vi "Digital - Continuous Output.vi"() -> ()   [LabVIEW 2020]
doc: "This example demonstrates how to continuously re-generate digital output data. That output is hardware timed, so each sample is output on the next tick of the sample clock.\n\nSome hardware (e.g. M Series DAQ) must use an external sample clock for digital tasks. To view a complete list of available sample clock sources, consult the Device Routes table in Measurement and Automation Explorer.\n\nFor instructions on how to connect your signals to the DAQ device, refer to your device documentation."
uses:
  <vilib>/Utility/error.llb/DialogType.ctl
  <vilib>/DAQmx/write.llb/DAQmx Write (Digital 1D U32 1Chan NSamp).vi
  <vilib>/DAQmx/create/channels.llb/DAQmx Create Channel (DO-Digital Output).vi
  <vilib>/DAQmx/configure/timing.llb/DAQmx Timing (Sample Clock).vi
  <vilib>/DAQmx/configure/trigger.llb/DAQmx Start Trigger (Digital Edge).vi
  <vilib>/DAQmx/configure/trigger.llb/DAQmx Start Trigger (Time).vi
  <vilib>/DAQmx/miscellaneous.llb/DAQmx Fill In Error Info.vi
  <resource>/objmgr/daqmx.rc
panel:
  in  "Frequency of Steps":dbl
  in  "Line(s)":tag="Dev1/port0/line0:7"
  in  "Stop":bool
  in  "Output Array":u32[](array[numeric])=[1, 2, 4, 8, 16, 32, 64, 128]
  in  "Trigger Type":T1(tab)
  in  "Edge":i32(ring)=10280 items=["Rising"=10280, "Falling"=10171]
  in  "Digital Trigger Source":tag="PFI1"
  in  "When":timestamp
  in  "Select Time\nManually":bool
  in  "Number of Samples":i32=1000
  in  "Sample Rate":dbl=1000.0
  in  "Sample Clock Source":tag="PFI0"
  out "Actual Sample Rate":dbl=1000.0 format="%0.2f"
  # "Channel Settings"
  # "Data to Write"
  # "Timing and Buffer Settings"
  # "Trigger Settings"
  # "To configure and use a start trigger you must have the necessary tab selected above.  Not all hardware supports triggering--refer to your device documentation for more info."
  # "If time is not manually set, task will begin after 10 seconds"
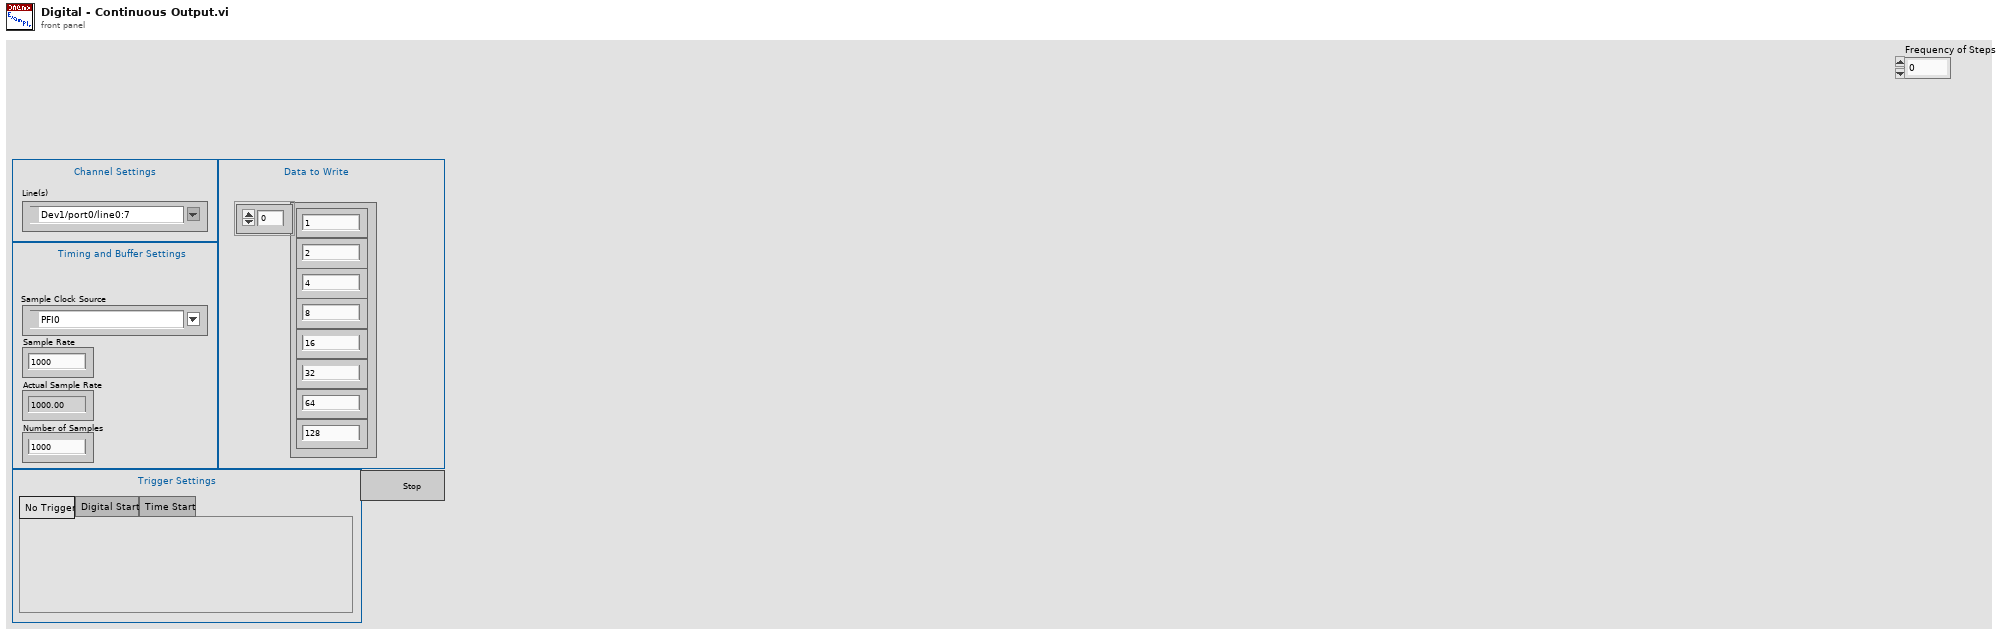
[diagram p1: front panel]
types:
  T1 = enum32{"No Trigger", "Digital Start", "Time Start"}
  T2 = typedef "DialogType.ctl" = u16
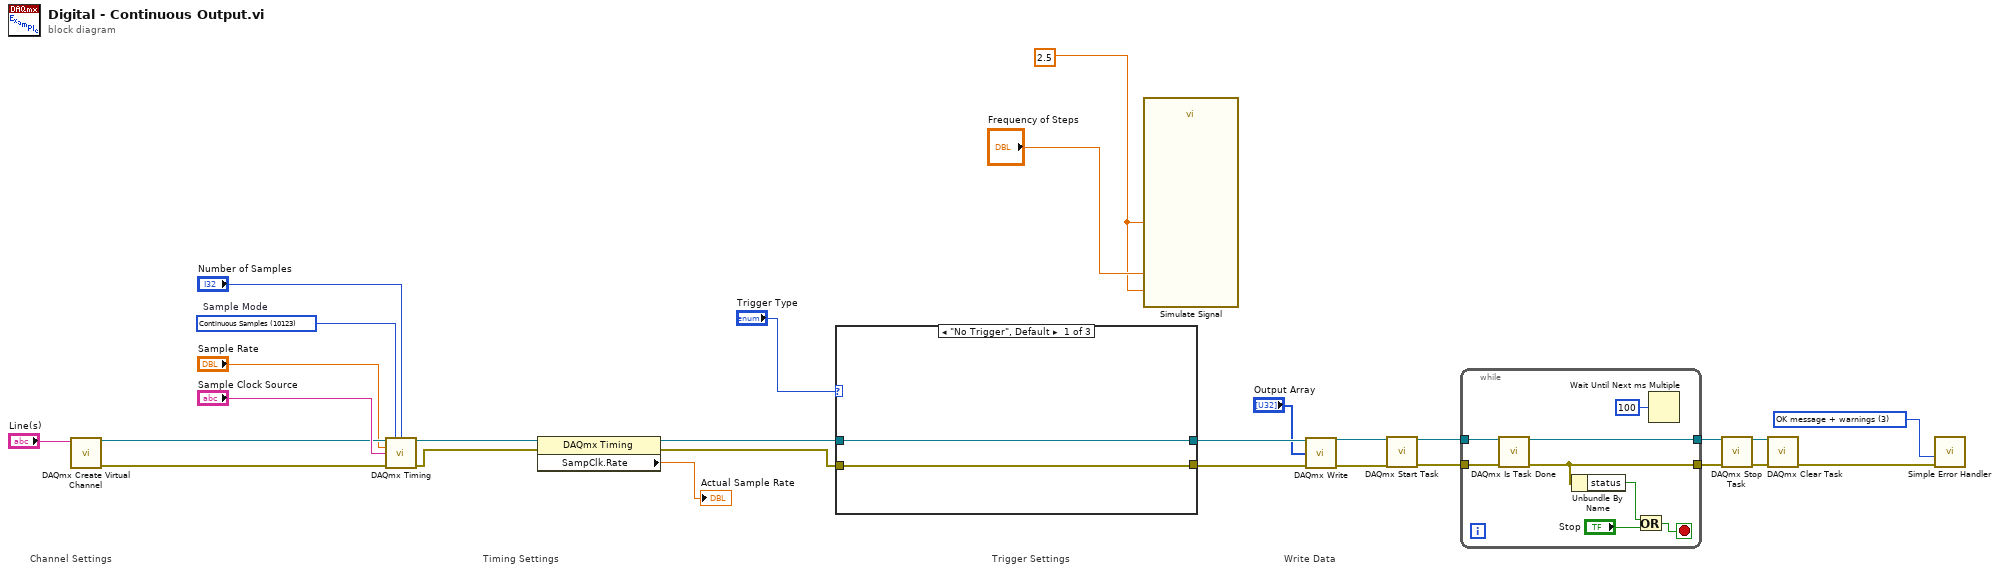
[diagram p0: block diagram]
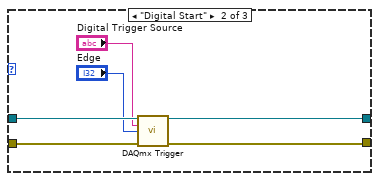
[diagram p2: hidden frame]
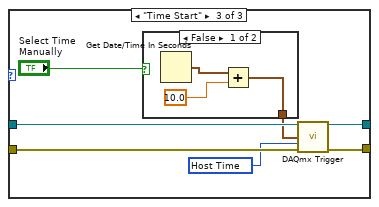
[diagram p3: hidden frame]
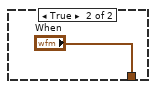
[diagram p4: hidden frame]
diagram:
  w1 = 2.5
  w3 = T2 3 items=["no dialog", "OK message", "continue or stop message", "OK message + warnings", "continue/stop + warnings"] ("type of dialog (OK msg:1)")
  w21 = 10123 items=["Finite Samples"=10178, "Continuous Samples"=10123, "Hardware Timed Single Point"=12522]  # Sample Mode
  # "Trigger Settings"
  # "Timing Settings"
  # "Write Data"
  # "Channel Settings"
  n1 = call-poly <vilib>:"DAQmx Create Virtual Channel.vi"("lines"="Line(s)") -> ("task out"=w25:refnum<k21>, "error out"=w24:errorcluster)  [unwired: 13 in]
  n2 = call-poly <vilib>:"DAQmx Timing.vi"("task/channels in"=w25, "sample mode"=w21, "samples per channel"="Number of Samples", "rate"="Sample Rate", "source"="Sample Clock Source", "error in"=w24) -> ("task out"=w20:refnum<k21>, "error out"=w19:errorcluster)  [unwired: 8 in]
  n3 = property class="DAQmx Timing"(reference=w20, error in=w19) -> (reference out=w17:refnum<k21>, error out=w16:errorcluster, "SampClk.Rate"=→"Actual Sample Rate":dbl)
  n4 = case shown="\"No Trigger\", Default" "Trigger Type" {
    tunnel: w17 -> [w30 w36 w43]
    tunnel: w16 -> [w29 w35 w42]
    tunnel: [w30 w34 w41] -> w15
    tunnel: [w29 w33 w40] -> w14
    frame "No Trigger", Default {
    }
    frame "Digital Start" {
      n5 = call-poly <vilib>:"DAQmx Trigger.vi"("task/channels in"=w36, "source"="Digital Trigger Source", "edge"="Edge", "error in"=w35) -> ("task out"=w34:refnum<k21>, "error out"=w33:errorcluster)  [unwired: 10 in]
    }
    frame "Time Start" {
      w37 = 16126 items=["Host Time"=16126, "I/O Device Time"=16127] ("timescale")
      n6 = case shown="False" "Select Time\nManually" {
        tunnel: [w45 "When"] -> w38
        frame False {
          n7 = Get Date/Time In Seconds() -> (seconds since 1Jan1904=w46:timestamp)
          n8 = Add(x=w46, y=10.0) -> (x+y=w45:timestamp)
        }
        frame True {
        }
      }
      n9 = call-poly <vilib>:"DAQmx Trigger.vi"("task/channels in"=w43, "when"=w38, "timescale"=w37, "error in"=w42) -> ("task out"=w41:refnum<k21>, "error out"=w40:errorcluster)  [unwired: 10 in]
    }
  }
  n10 = call "Simulate Signal"("Offset"=w1, "Frequency"="Frequency of Steps", "Amplitude"=w1) -> ()  [unwired: 11 in, 2 out]
  n11 = call-poly <vilib>:"DAQmx Write.vi"("task/channels in"=w15, "data"="Output Array", "error in"=w14) -> ("task out"=w12:refnum<k21>, "error out"=w11:errorcluster)  [unwired: 10 in, 1 out]
  n12 = call <vilib>:"DAQmx Start Task.vi"("task/channels in"=w12, "error in"=w11) -> ("task out"=w10:refnum<k21>, "error out"=w9:errorcluster)  [unwired: 12 in]
  n13 = while {
    tunnel: w10 -> [w55]
    tunnel: w9 -> [w54]
    tunnel: [w51] -> w4
    tunnel: [w53] -> w5
    stop <- w48 stop-if-true
    n14 = call <vilib>:"DAQmx Is Task Done.vi"("task/channels in"=w55, "error in"=w54) -> ("task out"=w53:refnum<k21>, "error out"=w51:errorcluster)  [unwired: 11 in, 1 out]
    n15 = Unbundle By Name(w51) -> ("status"=w50:bool)
    n16 = Or(x=w50, y="Stop") -> (x .or. y?=w48:bool)
    n17 = Wait Until Next ms Multiple(millisecond multiple=u32 100) -> ()  [unwired: 1 out]
  }
  n18 = call <vilib>:"DAQmx Stop Task.vi"("task/channels in"=w5, "error in"=w4) -> ("task out"=w7:refnum<k21>, "error out"=w6:errorcluster)  [unwired: 12 in]
  n19 = call <vilib>:"DAQmx Clear Task.vi"("task in"=w7, "error in"=w6) -> ("error out"=w28:errorcluster)  [unwired: 13 in]
  n20 = call <vilib>:"Simple Error Handler.vi"("type of dialog (OK msg:1)"=w3, "error in (no error)"=w28) -> ()  [unwired: 3 in, 5 out]
